vi "Rename Directory.vi"(8 "error in (no error)":errorcluster caption="错误输入（无错误）", 9 "NewPath":path, 10 "Path":path, 11 "FileSystem 输入":refnum<class "FileSystem.lvclass"> caption="DNL_LabVIEW Object in") -> (0 "error out":errorcluster caption="错误输出", 3 "FileSystem 输出":refnum<class "FileSystem.lvclass"> caption="DNL_LabVIEW Object out")   [LabVIEW 2011, in "FileSystem.lvclass"]
uses:
  FileSystem.lvclass
  Microsoft.VisualBasic
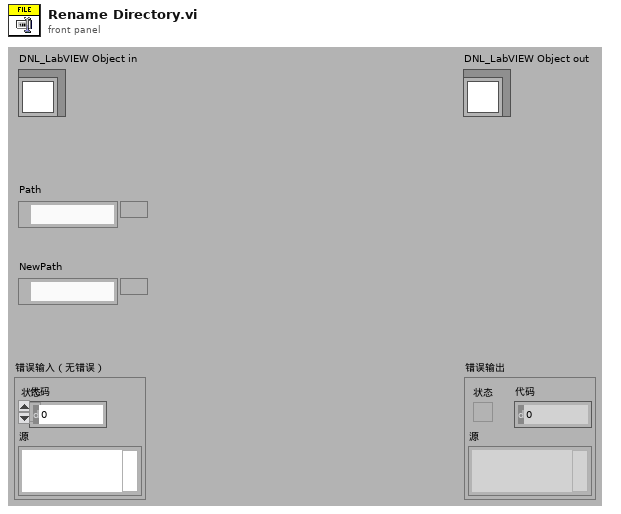
[diagram p1: front panel]
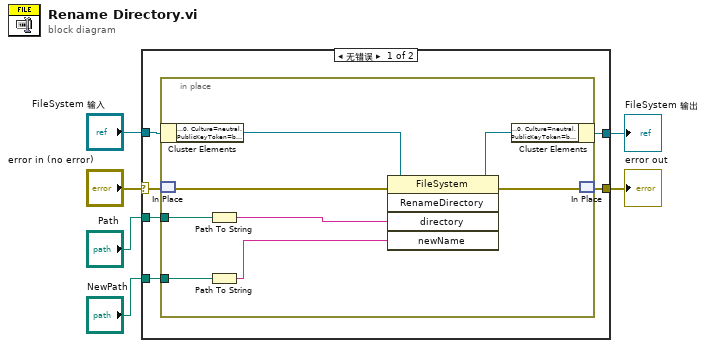
[diagram p0: block diagram]
diagram:
  n1 = case shown="无错误" "error in (no error)" {
    selector: "error in (no error)" -> [w10 w22]
    tunnel: [w9 w22] -> w5
    tunnel: [w11 w21] -> w3
    tunnel: "FileSystem 输入" -> [w12 w21]
    tunnel: "Path" -> [w8 _]
    tunnel: "NewPath" -> [w7 _]
    frame No Error {
      n2 = in-place {
        in-place-border: w8 -> [w18]
        in-place-border: w7 -> [w14]
        n3 = in-place-cluster #1(w12) -> ("FileSystem"=w20:refnum<k24>)
        n4 = in-place-match #2(w10) -> (w15:errorcluster)
        n5 = Path To String(path=w18) -> (string=w17:string)
        n6 = Path To String(path=w14) -> (string=w13:string)
        n7 = invoke class="FileSystem" method="RenameDirectory"(reference=w20, error in=w15, "directory"=w17, "newName"=w13) -> (reference out=w19:refnum<k24>, error out=w16:errorcluster)  [unwired: 1 in, 3 out]
        n8 = in-place-cluster #1("FileSystem"=w19) -> (w11:refnum<class "FileSystem.lvclass">)
        n9 = in-place-match #2(w16) -> (w9:errorcluster)
      }
    }
    frame Error {
    }
  }
  "error out" <- w5
  "FileSystem 输出" <- w3
